vi "TESTING COMMUNICATION.vi"() -> ()   [LabVIEW 2017]
uses:
  <vilib>/ethernetip/ethernetip.llb/EthernetIPSLC500FileType.ctl
  <vilib>/ethernetip/ethernetip.llb/EthernetIP SLC500 Read Float.vi
  <vilib>/ethernetip/ethernetip.llb/EthernetIP SLC500 Read Raw.vi
  <vilib>/ethernetip/ethernetip.llb/EthernetIP SLC500 Read Bit.vi
  <vilib>/ethernetip/ethernetip.lvlib
panel:
  out "Data 6":u8[](array[numeric]) format="%x"
  out "rejection":u8[](array[numeric]) format="%x"
  out "Data 4":u8[](array[numeric]) format="%x"
  out "Data 3":bool[](array[boolean])
  out "Data 2":bool[](array[boolean])
  out "(hi.lo) 3":u16
  out "rejection":u16
  out "count":u16
  in  "Number of Bytes":u32=1
  out "error out 3":errorcluster
  out "Data":u8[](array[numeric]) format="%x"
  out "error out":errorcluster
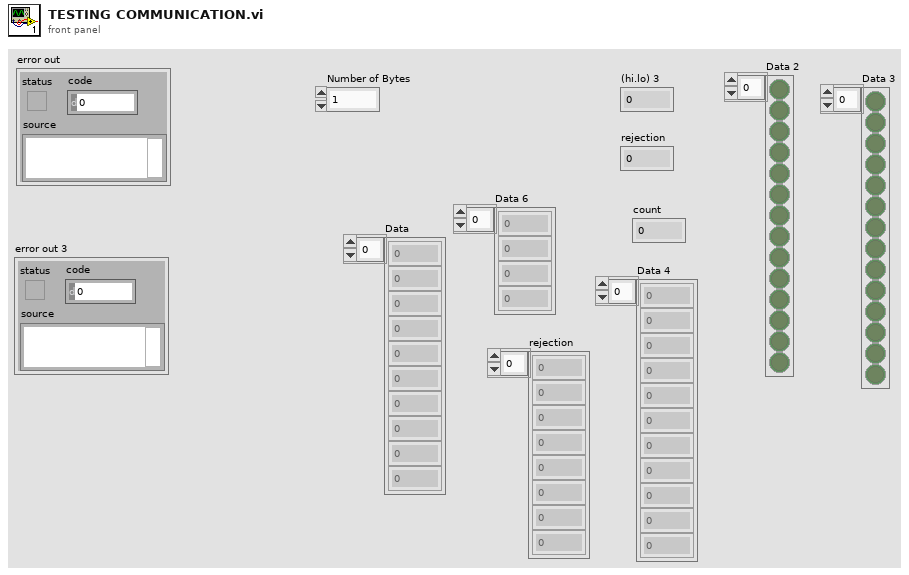
[diagram p1: front panel]
types:
  T1 = typedef "ethernetip.lvlib/EthernetIPSLC500FileType.ctl" = u8
  T2 = typedef "ethernetip.lvlib/ethernetip.ctl" = refnum<k21>
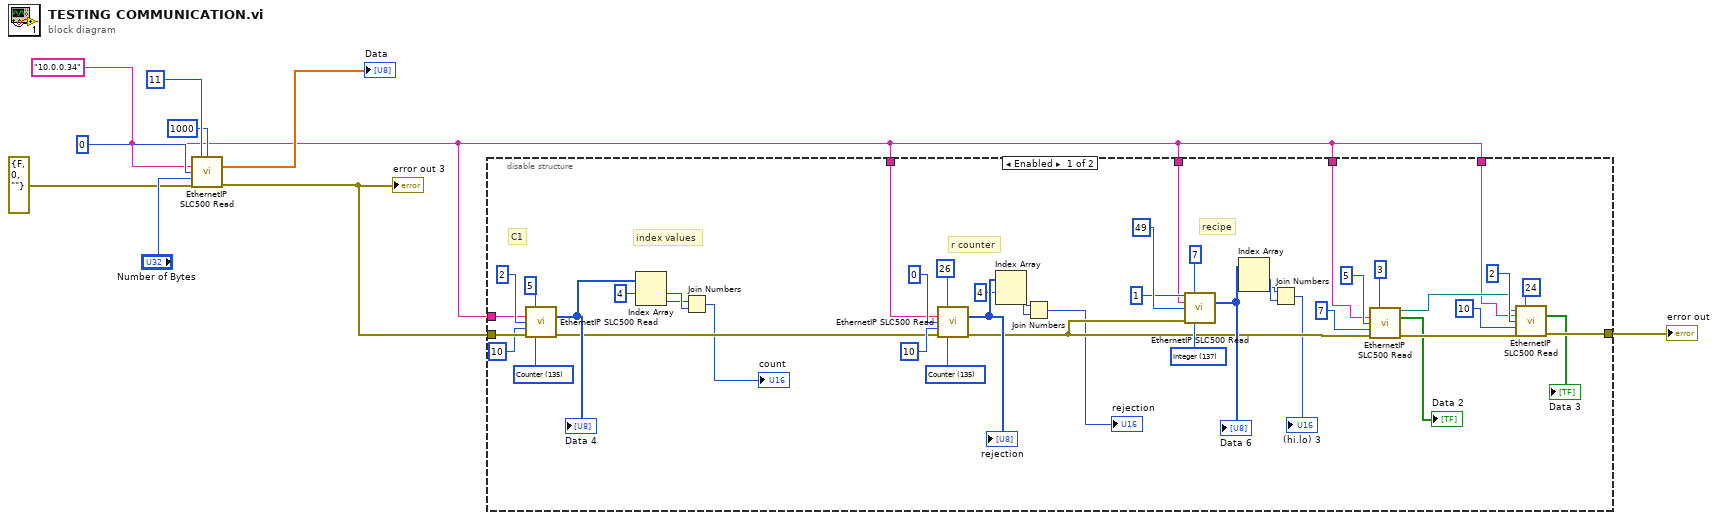
[diagram p0: block diagram]
diagram:
  w1 = "10.0.0.34" ("Network Path")
  n1 = call-poly <vilib>:"EthernetIP SLC500 Read.vi"("File Number"=u16 11, "Timeout (ms)"=1000, "Network Path"=w1, "Element Number"=u16 0, "Number of Elements"="Number of Bytes", "error in"=errorcluster {"status"=FALSE, "code"=0, "source"=""}) -> ("Data"=→"Data":sgl[], "error out"=w4:errorcluster)  [unwired: 7 in, 1 out]
  "error out 3" <- w4
  n2 = disable-structure shown="Enabled" {
    disable-tunnel: w4 -> [w54 w55]
    disable-tunnel: [w23 w55] -> w8
    disable-tunnel: w1 -> [w21 _]
    disable-tunnel: w1 -> [w20 _]
    disable-tunnel: w1 -> [w19 _]
    disable-tunnel: w1 -> [w18 _]
    disable-tunnel: w1 -> [w17 _]
    frame Enabled {
      w37 = T1 137 items=["Status"=132, "Bit"=133, "Timer"=134, "Counter"=135, "Control"=136, "Integer"=137, "Float"=138, "Output"=139, "Input"=140, "String"=141, "ASCII"=142] ("File Type")
      w41 = T1 135 items=["Status"=132, "Bit"=133, "Timer"=134, "Counter"=135, "Control"=136, "Integer"=137, "Float"=138, "Output"=139, "Input"=140, "String"=141, "ASCII"=142] ("File Type")
      w52 = T1 135 items=["Status"=132, "Bit"=133, "Timer"=134, "Counter"=135, "Control"=136, "Integer"=137, "Float"=138, "Output"=139, "Input"=140, "String"=141, "ASCII"=142] ("File Type")
      # "index values"
      # "recipe"
      # "r counter"
      # "C1"
      n3 = call-poly <vilib>:"EthernetIP SLC500 Read.vi"("File Number"=u16 5, "Network Path"=w19, "Element Number"=u16 2, "Number of Bytes"=u32 10, "error in"=w54, "File Type"=w52) -> ("Data"=w49:u8[], "error out"=w39:errorcluster)  [unwired: 7 in, 1 out]
      "Data 4" <- w49
      n4 = Index Array(array=w49, index #1=4 ("index")) -> (element #1=w48:u8, element #2=w47:u8)  [unwired: 1 in]
      n5 = Join Numbers(hi=w47, lo=w48) -> ((hi.lo)=→"count":u16)
      n6 = call-poly <vilib>:"EthernetIP SLC500 Read.vi"("File Number"=u16 26, "Network Path"=w20, "Element Number"=u16 0, "Number of Bytes"=u32 10, "error in"=w39, "File Type"=w41) -> ("Data"=w44:u8[], "error out"=w28:errorcluster)  [unwired: 7 in, 1 out]
      "rejection" <- w44
      n7 = Index Array(array=w44, index #1=4 ("index")) -> (element #1=w45:u8, element #2=w46:u8)  [unwired: 1 in]
      n8 = Join Numbers(hi=w46, lo=w45) -> ((hi.lo)=→"rejection":u16)
      n9 = call-poly <vilib>:"EthernetIP SLC500 Read.vi"("File Number"=u16 7, "Network Path"=w21, "Element Number"=u16 49, "Number of Bytes"=u32 1, "error in"=w28, "File Type"=w37) -> ("Data"=w35:u8[])  [unwired: 7 in, 2 out]
      "Data 6" <- w35
      n10 = Index Array(array=w35) -> (element #1=w34:u8, element #2=w33:u8)  [unwired: 2 in]
      n11 = Join Numbers(hi=w33, lo=w34) -> ((hi.lo)=→"(hi.lo) 3":u16)
      n12 = call-poly <vilib>:"EthernetIP SLC500 Read.vi"("File Number"=u16 3, "Network Path"=w18, "Element Number"=u16 5, "Number of Bits"=u32 7 ("Number of Bytes"), "error in"=w28) -> ("Session out"=w22:T2, "Data"=→"Data 2":bool[], "error out"=w25:errorcluster)  [unwired: 8 in]
      n13 = call-poly <vilib>:"EthernetIP SLC500 Read.vi"("Session in"=w22, "File Number"=u16 24, "Network Path"=w17, "Element Number"=u16 2, "Number of Bits"=u32 10 ("Number of Bytes"), "error in"=w25) -> ("Data"=→"Data 3":bool[], "error out"=w23:errorcluster)  [unwired: 7 in, 1 out]
    }
    frame Disabled {
    }
  }
  "error out" <- w8
